vi "zest_5_part_1.vi"() -> ()   [LabVIEW 2023]
panel:
  out "Array":bool[](array[boolean])
  in  "stop":bool
  in  "operation":enum16{"AND", "OR", "XOR"}(ring)
  out "Boolean 24":bool
  out "Boolean 23":bool
  out "Boolean 22":bool
  out "Boolean 21":bool
  out "Boolean 20":bool
  out "Boolean 19":bool
  out "Boolean 18":bool
  out "Boolean 17":bool
  in  "Boolean 16":bool
  in  "Boolean 15":bool
  in  "Boolean 14":bool
  in  "Boolean 13":bool
  in  "Boolean 12":bool
  in  "Boolean 11":bool
  in  "Boolean 10":bool
  in  "Boolean 9":bool
  in  "Boolean 8":bool
  in  "Boolean 7":bool
  in  "Boolean 6":bool
  in  "Boolean 5":bool
  in  "Boolean 4":bool
  in  "Boolean 3":bool
  in  "Boolean 2":bool
  in  "Boolean":bool
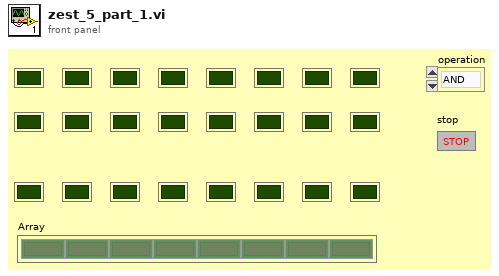
[diagram p1: front panel]
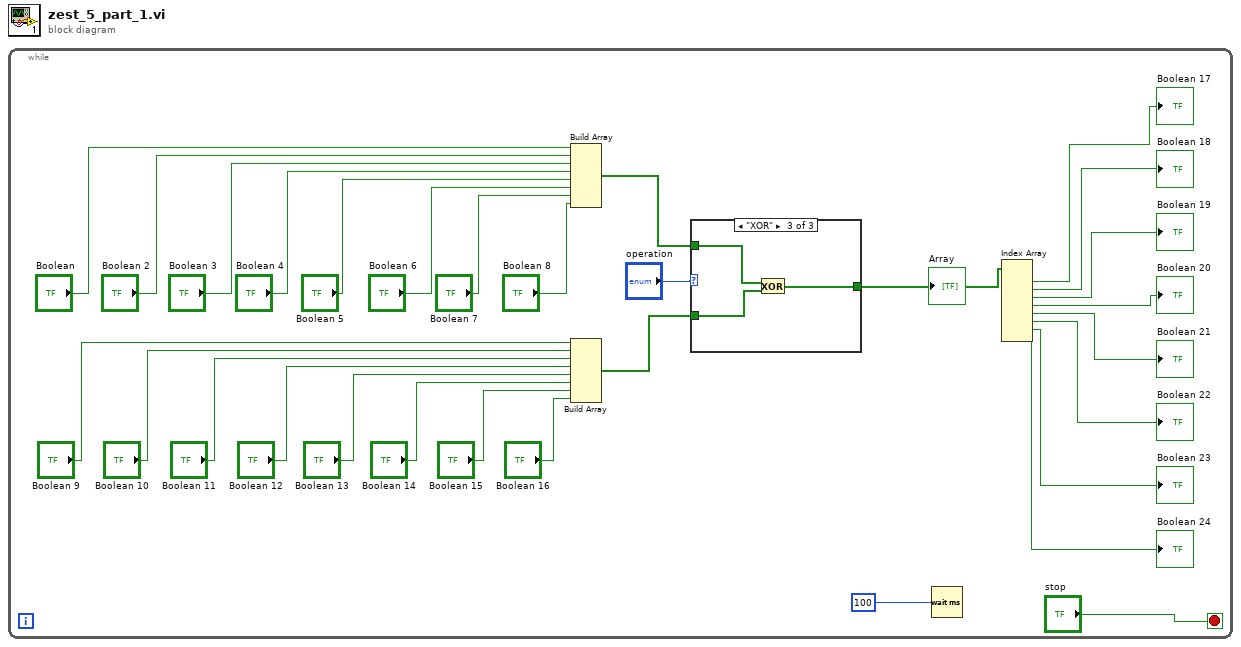
[diagram p0: block diagram]
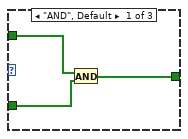
[diagram p2: hidden frame]
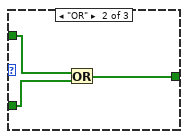
[diagram p3: hidden frame]
diagram:
  n1 = while {
    stop <- "stop" stop-if-true
    n2 = Build Array("Boolean", "Boolean 2", "Boolean 3", "Boolean 4", "Boolean 5", "Boolean 6", "Boolean 7", "Boolean 8") -> (w12:bool[])
    n3 = Build Array("Boolean 9", "Boolean 10", "Boolean 11", "Boolean 12", "Boolean 13", "Boolean 14", "Boolean 15", "Boolean 16") -> (w13:bool[])
    n4 = case shown="\"XOR\"" "operation" {
      tunnel: w13 -> [w32 w36 w38]
      tunnel: w12 -> [w33 w35 w39]
      tunnel: [w31 w34 w37] -> w11
      frame "AND", Default {
        n5 = And(x=w33, y=w32) -> (x .and. y?=w31:bool[])
      }
      frame "OR" {
        n6 = Or(x=w35, y=w36) -> (x .or. y?=w34:bool[])
      }
      frame "XOR" {
        n7 = Exclusive Or(1:w38, 2:w39) -> (0:w37:bool[])
      }
    }
    "Array" <- w11
    n8 = Wait (ms)(milliseconds to wait=100) -> ()  [unwired: 1 out]
    n9 = Index Array(array=w11) -> (element #1=→"Boolean 17":bool, element #2=→"Boolean 18":bool, element #3=→"Boolean 19":bool, element #4=→"Boolean 20":bool, element #5=→"Boolean 21":bool, element #6=→"Boolean 22":bool, element #7=→"Boolean 23":bool, element #8=→"Boolean 24":bool)  [unwired: 8 in]
  }
